vi "Configure Acquisition.vi"(0 "RedPitaya connection in":refnum<k5>, 1 "Decimation/Sampling Rate":enum16{"", "Sampling rate", "Decimation"}(ring), 2 "Sampling Rate":T1(ring), 3 "Decimation":u32(ring) items=["65536"=65536, "8192"=8192, "1024"=1024, "64"=64, "8"=8, "1"=1], 4 "Averaging":enum16{"None", "AVG ON", "AVG OFF"}(ring), 5 "error in":errorcluster, 12 "timeout ms (2000)":i32=2000) -> (14 "RedPitaya connection out":refnum<k5>, 19 "error out":errorcluster)   [LabVIEW 2010, in "RedPitaya.lvlib"]
doc: "Configures the propertise of acquisition. To set acquisition decimation or sampling rate first select which you want to set by input <b>Decimation/Sampling Rate</b>."
uses:
  RedPitaya.lvlib
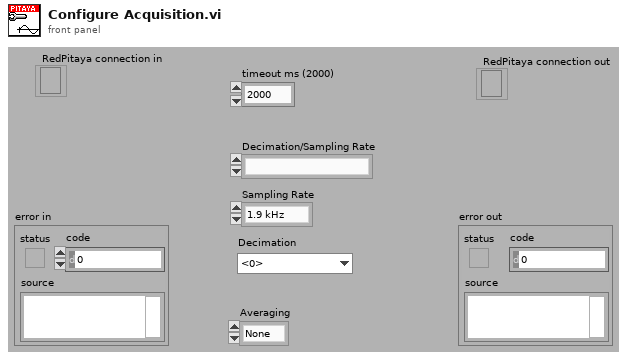
[diagram p1: front panel]
types:
  T1 = enum16{"1.9 kHz", "15.2 kHz", "103.8 kHz", "1.9 MHZ", "15.6 MHz", "125 MHz"}
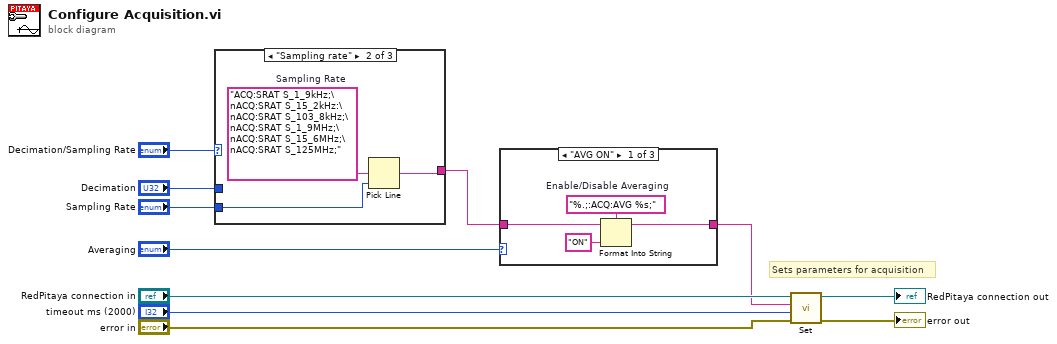
[diagram p0: block diagram]
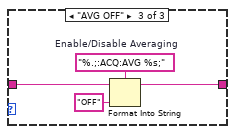
[diagram p3: hidden frame]
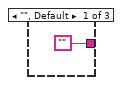
[diagram p4: hidden frame]
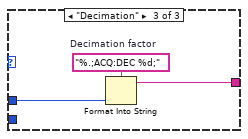
[diagram p5: hidden frame]
diagram:
  # "Sets parameters for acquisition"
  n1 = case shown="\"Sampling rate\"" "Decimation/Sampling Rate" {
    tunnel: ["" w14 w17] -> w11
    tunnel: "Decimation" -> [_ _ w16]
    tunnel: "Sampling Rate" -> [_ w13 _]
    frame "", Default {
    }
    frame "Sampling rate" {
      w15 = "ACQ:SRAT S_1_9kHz;\nACQ:SRAT S_15_2kHz:\nACQ:SRAT S_103_8kHz;\nACQ:SRAT S_1_9MHz;\nACQ:SRAT S_15_6MHz;\nACQ:SRAT S_125MHz;"  # Sampling Rate
      n2 = Pick Line(multi-line string=w15, line index=w13) -> (output string=w14:string)  [unwired: 1 in]
    }
    frame "Decimation" {
      w18 = "%.;ACQ:DEC %d;"  # Decimation factor
      n3 = Format Into String(format string=w18, w16) -> (resulting string=w17:string)  [unwired: 2 in, 1 out]
    }
  }
  n4 = case shown="\"AVG ON\"" "Averaging" {
    tunnel: [w22 w23 w27] -> w9
    tunnel: w11 -> [w21 w23 w26]
    frame "AVG ON" {
      w20 = "%.;:ACQ:AVG %s;"  # Enable/Disable Averaging
      n5 = Format Into String(format string=w20, initial string=w21, "ON") -> (resulting string=w22:string)  [unwired: 1 in, 1 out]
    }
    frame "None", Default {
    }
    frame "AVG OFF" {
      w25 = "%.;:ACQ:AVG %s;"  # Enable/Disable Averaging
      n6 = Format Into String(format string=w25, initial string=w26, "OFF") -> (resulting string=w27:string)  [unwired: 1 in, 1 out]
    }
  }
  n7 = call "Set.vi"("error in"="error in", "timeout ms (2000)"="timeout ms (2000)", "SCPI Message"=w9, "RedPitaya connection in"="RedPitaya connection in") -> ("error out"=→"error out":errorcluster, "RedPitaya connection out"=→"RedPitaya connection out":refnum<k5>)  [unwired: 5 in, 1 out]
